vi "Del - UDP Data Link - Configuration Utilities - Remove Old Tx Channels.vi"(8 "error in (no error)":errorcluster, 11 "Device Item Ref in":T1 format="%.0x") -> (0 "error out":errorcluster, 2 "Tx Dependent Refs":T1[](array[typedef]) format="%.0x", 3 "Device Item Ref out":T1 format="%.0x")   [LabVIEW 2016, in "UDP-Custom-Device System Explorer.lvlib"]
uses:
  UDP-Custom-Device System Explorer.lvlib
  <vilib>/NI Veristand/Custom Device API/Custom Device Item Ref.ctl
  Shared/Constants.vi
  <vilib>/NI Veristand/Custom Device Tools/Custom Device Utility Library/NI VeriStand - Search for Item by GUID.vi
  <vilib>/NI Veristand/Custom Device API/Get Item Property (String Array).vi
  <vilib>/NI Veristand/Custom Device API/Set Item Property (String Array).vi
  <vilib>/NI VeriStand/Custom Device Tools/Custom Device Utility Library/Custom Device Utility Library.lvlib
  <vilib>/NI VeriStand/Custom Device API/Custom Device API.lvlib
  Shared/UDP-Custom-Device Shared.lvlib
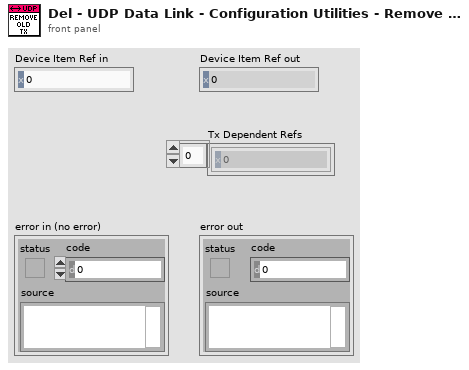
[diagram p1: front panel]
types:
  T1 = typedef "Custom Device API.lvlib/Custom Device Item Ref.ctl" = u64
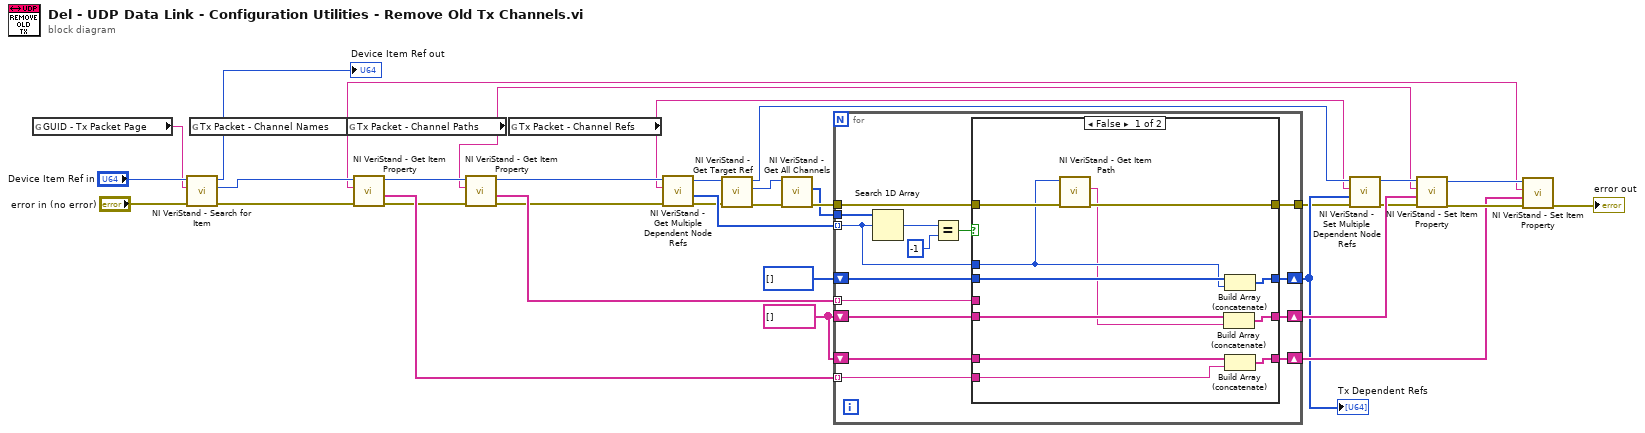
[diagram p0: block diagram]
diagram:
  w22 = string[] []
  n1 = global read "Constants.vi" "GUID - Tx Packet Page"() -> (w4:string)
  n2 = call-poly <vilib>:"NI VeriStand - Search for Item.vi"("error in"="error in (no error)", "Item GUID"=w4, "Section Ref in"="Device Item Ref in") -> ("error out"=w14:errorcluster, "Item Ref"=w16:T1, "Section Ref out"=→"Device Item Ref out":T1)  [unwired: 5 in, 1 out]
  n3 = global read "Constants.vi" "Tx Packet - Channel Names"() -> (w3:string)
  n4 = global read "Constants.vi" "Tx Packet - Channel Paths"() -> (w2:string)
  n5 = call-poly <vilib>:"NI VeriStand - Get Item Property.vi"("error in (no error)"=w14, "Property Name"=w3, "Item Ref in"=w16) -> ("error out"=w15:errorcluster, "Value"=w20:string[], "Item Ref out"=w17:T1)  [unwired: 5 in, 1 out]
  n6 = call-poly <vilib>:"NI VeriStand - Get Item Property.vi"("error in (no error)"=w15, "Property Name"=w2, "Item Ref in"=w17) -> ("error out"=w19:errorcluster, "Value"=w21:string[], "Item Ref out"=w18:T1)  [unwired: 5 in, 1 out]
  n7 = global read "Constants.vi" "Tx Packet - Channel Refs"() -> (w1:string)
  n8 = call <vilib>:"NI VeriStand - Get Multiple Dependent Node Refs.vi"("error in (no error)"=w19, "Base Property Name"=w1, "Item Ref in"=w18) -> ("error out"=w7:errorcluster, "Dependent Node Refs"=w12:T1[], "Item Ref out"=w9:T1)  [unwired: 6 in]
  n9 = call <vilib>:"NI VeriStand - Get Target Ref.vi"("error in"=w7, "Item Ref in"=w9) -> ("error out"=w8:errorcluster, "Target Ref"=w10:T1, "Item Ref out"=w25:T1)  [unwired: 6 in, 1 out]
  n10 = call <vilib>:"NI VeriStand - Get All Channels.vi"("error in"=w8, "Section Ref in"=w10) -> ("error out"=w13:errorcluster, "Channel Refs"=w11:T1[])  [unwired: 6 in, 2 out]
  n11 = for {
    tunnel: w11 -> [w49]
    tunnel: w12 -> [w36] mode=indexing
    tunnel: w13 -> [w45]
    tunnel: w20 -> [w44] mode=indexing
    tunnel: w21 -> [w43] mode=indexing
    shift-right: [w38] -> w29
    shift-left: w22 -> [w41]
    shift-right: [w37] -> w30
    shift-left: w22 -> [w42]
    shift-right: [w39] -> w26
    shift-left: T1[] [] -> [w40]
    tunnel: [w35] -> w24
    n12 = Search 1D Array(1D array=w49, element=w36) -> (index of element=w48:i32)  [unwired: 1 in]
    n13 = Equal?(x=w48, y=-1) -> (x = y?=w46:bool)
    n14 = case shown="False" w46 {
      tunnel: w45 -> [w53 w61]
      tunnel: w44 -> [w55 _]
      tunnel: w43 -> [_ _]
      tunnel: w42 -> [w56 w62]
      tunnel: w41 -> [w58 w63]
      tunnel: w40 -> [w60 w64]
      tunnel: [w59 w64] -> w39
      tunnel: [w57 w63] -> w38
      tunnel: [w54 w62] -> w37
      tunnel: w36 -> [w51 _]
      tunnel: [w52 w61] -> w35
      frame False {
        n15 = call <vilib>:"NI VeriStand - Get Item Path.vi"("error in (no error)"=w53, "Item Ref in"=w51) -> ("error out"=w52:errorcluster, "Path"=w50:string)  [unwired: 6 in, 2 out]
        n16 = Build Array (concatenate)(w58, w50) -> (w57:string[])
        n17 = Build Array (concatenate)(w60, w51) -> (w59:T1[])
        n18 = Build Array (concatenate)(w56, w55) -> (w54:string[])
      }
      frame True {
      }
    }
  }
  "Tx Dependent Refs" <- w26
  n19 = call <vilib>:"NI VeriStand - Set Multiple Dependent Node Refs.vi"("error in (no error)"=w24, "Dependent Node Refs"=w26, "Base Property Name"=w1, "Item Ref in"=w25) -> ("error out"=w27:errorcluster, "Item Ref out"=w28:T1)  [unwired: 6 in]
  n20 = call-poly <vilib>:"NI VeriStand - Set Item Property.vi"("error in (no error)"=w27, "Value"=w29, "Property Name"=w2, "Item Ref in"=w28) -> ("error out"=w31:errorcluster, "Item Ref out"=w32:T1)  [unwired: 5 in, 1 out]
  n21 = call-poly <vilib>:"NI VeriStand - Set Item Property.vi"("error in (no error)"=w31, "Value"=w30, "Property Name"=w3, "Item Ref in"=w32) -> ("error out"=→"error out":errorcluster)  [unwired: 5 in, 2 out]
